vi "Read back eight floats from csv file.vi"(0 "File Path":path, 11 "error in (no error)":errorcluster) -> (2 "item 1":dbl, 3 "item 2":dbl, 4 "item 3":dbl, 6 "item 4":dbl, 8 "item 5":dbl, 10 "item 6":dbl, 13 "item 8":dbl, 14 "item 7":dbl, 15 "error out":errorcluster)   [LabVIEW 2013]
uses:
  <vilib>/Utility/file.llb/Read From Spreadsheet File (string).vi
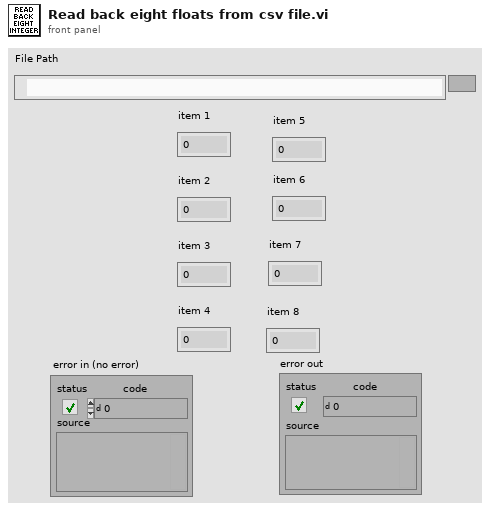
[diagram p1: front panel]
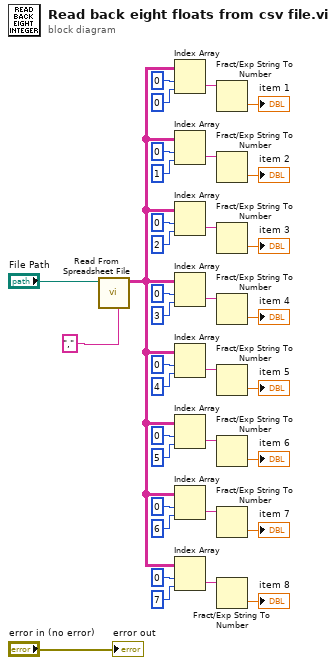
[diagram p0: block diagram]
diagram:
  n1 = call-poly <vilib>:"Read From Spreadsheet File.vi"("delimiter (\\t)"="," ("delimiter (\\t)"), "file path (dialog if empty)"="File Path") -> ("all rows"=w18:string[][])  [unwired: 5 in, 4 out]
  n2 = Index Array(array=w18, index (row)=0, index (col)=0 ("disabled index (col)")) -> (element=w16:string)
  n3 = Index Array(array=w18, index (row)=0, index (col)=1 ("disabled index (col)")) -> (element=w14:string)
  n4 = Index Array(array=w18, index (row)=0, index (col)=2 ("disabled index (col)")) -> (element=w12:string)
  n5 = Index Array(array=w18, index (row)=0, index (col)=3 ("disabled index (col)")) -> (element=w10:string)
  n6 = Index Array(array=w18, index (row)=0, index (col)=4 ("disabled index (col)")) -> (element=w8:string)
  n7 = Index Array(array=w18, index (row)=0, index (col)=5 ("disabled index (col)")) -> (element=w6:string)
  n8 = Index Array(array=w18, index (row)=0, index (col)=6 ("disabled index (col)")) -> (element=w4:string)
  n9 = Index Array(array=w18, index (row)=0, index (col)=7 ("disabled index (col)")) -> (element=w2:string)
  n10 = Fract/Exp String To Number(string=w16) -> (number=→"item 1":dbl)  [unwired: 3 in, 1 out]
  n11 = Fract/Exp String To Number(string=w14) -> (number=→"item 2":dbl)  [unwired: 3 in, 1 out]
  n12 = Fract/Exp String To Number(string=w12) -> (number=→"item 3":dbl)  [unwired: 3 in, 1 out]
  n13 = Fract/Exp String To Number(string=w10) -> (number=→"item 4":dbl)  [unwired: 3 in, 1 out]
  n14 = Fract/Exp String To Number(string=w8) -> (number=→"item 5":dbl)  [unwired: 3 in, 1 out]
  n15 = Fract/Exp String To Number(string=w6) -> (number=→"item 6":dbl)  [unwired: 3 in, 1 out]
  n16 = Fract/Exp String To Number(string=w4) -> (number=→"item 7":dbl)  [unwired: 3 in, 1 out]
  n17 = Fract/Exp String To Number(string=w2) -> (number=→"item 8":dbl)  [unwired: 3 in, 1 out]
  "error out" <- "error in (no error)"
